vi "Autonomous Independent.vi"   [LabVIEW 2017]
doc: "This VI is called when autonomous begins, and will automatically be terminated when autonomous ends. You can carry out timed or sensor driven robot movement independently without needing to return to the caller."
uses:
  <vilib>/Rock Robotics/Network Tables/NT Read String.vi
  Robot Global Data.vi
  <vilib>/Rock Robotics/Network Tables/NT Write String.vi
  <vilib>/Rock Robotics/WPI/ThirdParty/Sensors/ADIS16448 IMU/ADIS16448_IMU.lvlib
types:
  T1 = typedef "ADIS16448_IMU.lvlib/ADI_IMU_ADIS16448_IMUDevRef.ctl" = cluster{"DevStatus":errorcluster, "Handle":i32, "SPI Bus":T2, "Device Found":bool, "Device Ready":bool, "Yaw Axis":enum16{"X", "Y", "Z"}, "AHRS Algorithm":enum16{"Complementary", "Madgwick"}, "Serial":u16, "Lot ID 2":u16, "Lot ID 1":u16, "Bytes Per Sample":u16, "Calibrate On Open?":bool}
  T2 = typedef "spi_bus.ctl" = enum16{"SPI On-Board, CS0", "SPI On-Board, CS1", "SPI On-Board, CS2", "SPI On-Board, CS3", "SPI MXP", "Invalid"}
  T3 = cluster{"X Angle":dbl, "Y Angle":dbl, "Z Angle":dbl}
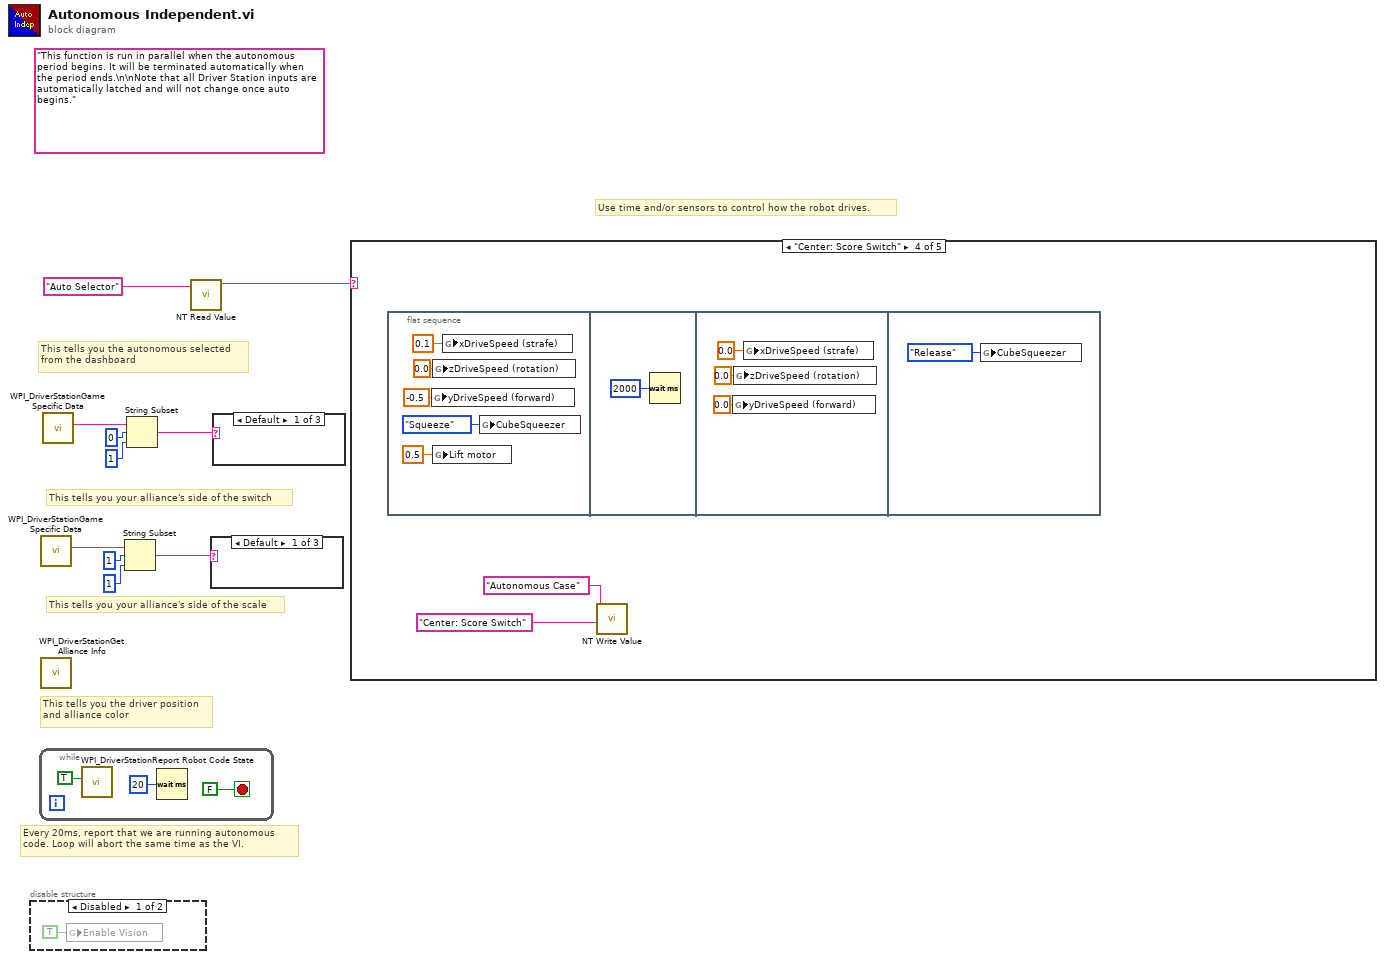
[diagram p0: block diagram]
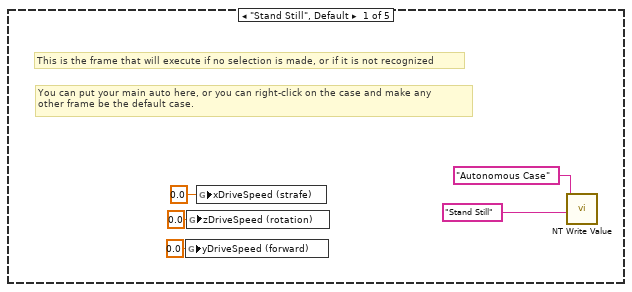
[diagram p7: hidden frame]
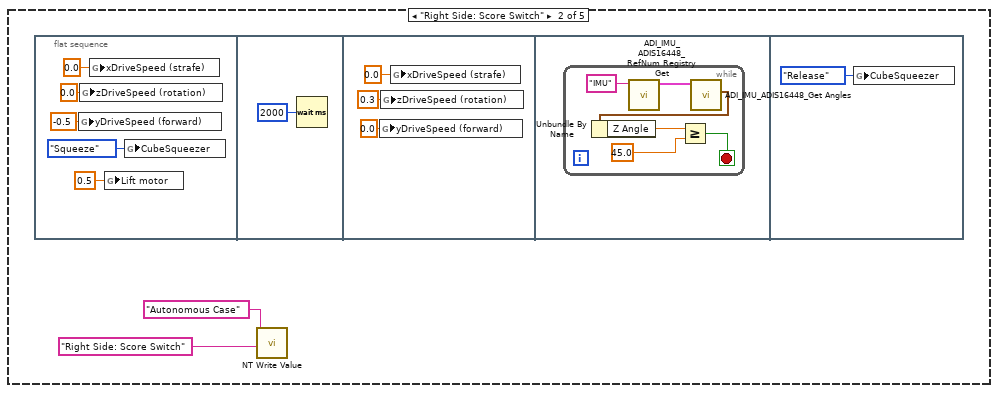
[diagram p8: hidden frame]
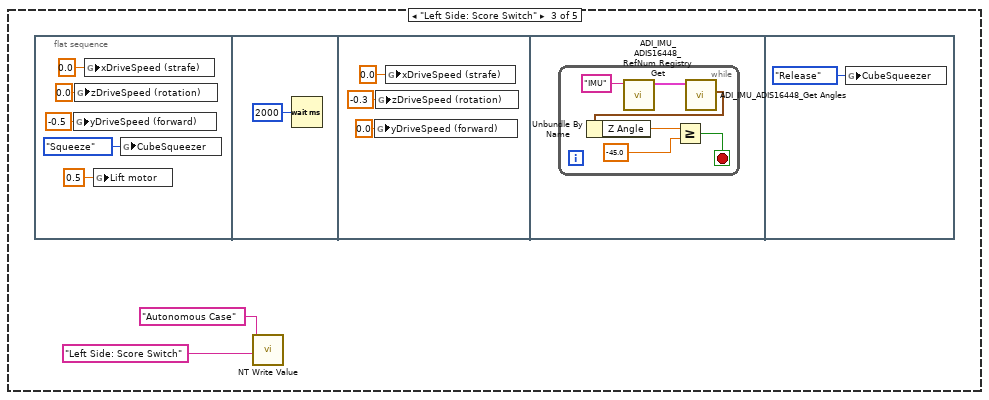
[diagram p9: hidden frame]
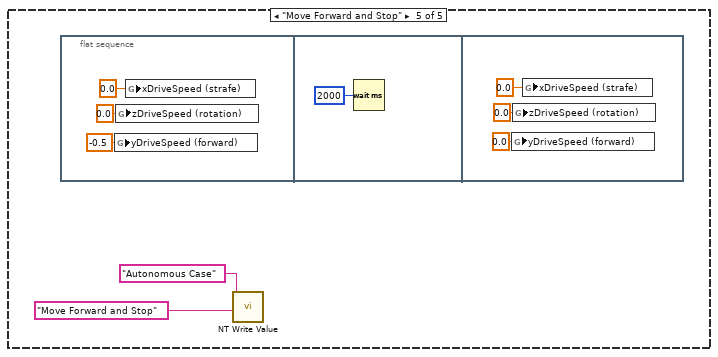
[diagram p10: hidden frame]
diagram:
  (unwired) "This function is run in parallel when the autonomous period begins. It will be terminated automatically when the period ends.\n\nNote that all Driver Station inputs are automatically latched and will not change once auto begins."
  # "This tells you your alliance's side of the scale"
  # "This tells you your alliance's side of the switch"
  # "This tells you the autonomous selected\nfrom the dashboard"
  # "Every 20ms, report that we are running autonomous\ncode. Loop will abort the same time as the VI."
  # "Use time and/or sensors to control how the robot drives."
  # "This tells you the driver position\nand alliance color"
  n1 = disable-structure shown="Disabled" {
    frame Disabled {
      n2 = global write "Robot Global Data.vi" "Enable Vision"(TRUE ("Enable Vision")) -> ()
    }
    frame Enabled {
    }
  }
  n3 = while {
    stop <- FALSE stop-if-true
    n4 = call <vilib>:"WPI_DriverStationReport Robot Code State.vi"("Autonomous"=TRUE) -> ()  [unwired: 10 in, 1 out]
    n5 = Wait (ms)(milliseconds to wait=u32 20) -> ()  [unwired: 1 out]
  }
  n6 = call <vilib>:"WPI_DriverStationGame Specific Data.vi"() -> ("Game Specific Data"=w5:string)  [unwired: 11 in]
  n7 = call <vilib>:"WPI_DriverStationGet Alliance Info.vi"() -> ()  [unwired: 12 out]
  n8 = call <vilib>:"WPI_DriverStationGame Specific Data.vi"() -> ("Game Specific Data"=w8:string)  [unwired: 11 in]
  n9 = String Subset(string=w5, offset (0)=1, length (rest)=1 ("length (rest)")) -> (substring=w3:string)
  n10 = String Subset(string=w8, offset (0)=0, length (rest)=1 ("length (rest)")) -> (substring=w6:string)
  n11 = call-poly <vilib>:"NT Read Value.vi"("Name"="Auto Selector") -> ("String"=w9:string)  [unwired: 9 in, 1 out]
  n12 = case shown="Default" w3 {
    frame Default {
    }
    frame "L" {
    }
    frame "R" {
    }
  }
  n13 = case shown="Default" w6 {
    frame Default {
    }
    frame "L" {
    }
    frame "R" {
    }
  }
  n14 = case shown="\"Center: Score Switch\"" w9 {
    frame "Stand Still", Default {
      # "You can put your main auto here, or you can right-click on the case and make any\nother frame be the default case."
      # "This is the frame that will execute if no selection is made, or if it is not recognized"
      n15 = global write "Robot Global Data.vi" "yDriveSpeed (forward)"(0.0 ("xDriveSpeed (strafe)")) -> ()
      n16 = global write "Robot Global Data.vi" "zDriveSpeed (rotation)"(0.0 ("xDriveSpeed (strafe)")) -> ()
      n17 = global write "Robot Global Data.vi" "xDriveSpeed (strafe)"(0.0 ("xDriveSpeed (strafe)")) -> ()
      n18 = call-poly <vilib>:"NT Write Value.vi"("String"="Stand Still", "Name"="Autonomous Case") -> ()  [unwired: 9 in, 1 out]
    }
    frame "Right Side: Score Switch" {
      n19 = flat-sequence {
        frame #0 {
          n20 = global write "Robot Global Data.vi" "yDriveSpeed (forward)"(-0.5 ("xDriveSpeed (strafe)")) -> ()
          n21 = global write "Robot Global Data.vi" "zDriveSpeed (rotation)"(0.0 ("xDriveSpeed (strafe)")) -> ()
          n22 = global write "Robot Global Data.vi" "xDriveSpeed (strafe)"(0.0 ("xDriveSpeed (strafe)")) -> ()
          n23 = global write "Robot Global Data.vi" "Lift motor"(0.5 ("Lift motor")) -> ()
          n24 = global write "Robot Global Data.vi" "CubeSqueezer"(enum16{"Squeeze", "Release"}."Squeeze" ("CubeSqueezer")) -> ()
        }
        frame #1 {
          n25 = Wait (ms)(milliseconds to wait=u32 2000) -> ()  [unwired: 1 out]
        }
        frame #2 {
          n26 = global write "Robot Global Data.vi" "yDriveSpeed (forward)"(0.0 ("xDriveSpeed (strafe)")) -> ()
          n27 = global write "Robot Global Data.vi" "zDriveSpeed (rotation)"(0.3 ("xDriveSpeed (strafe)")) -> ()
          n28 = global write "Robot Global Data.vi" "xDriveSpeed (strafe)"(0.0 ("xDriveSpeed (strafe)")) -> ()
        }
        frame #3 {
          n29 = while {
            stop <- w31 stop-if-true
            n30 = call <vilib>:"ADI_IMU_ADIS16448_RefNum Registry Get.vi"("refnum name"="IMU") -> ("ADI IMU DevRef"=w35:T1)  [unwired: 9 in, 1 out]
            n31 = call <vilib>:"ADI_IMU_ADIS16448_Get Angles.vi"("ADI IMU DevRef"=w35) -> ("IMU Angles Out"=w34:T3)  [unwired: 7 in, 3 out]
            n32 = Unbundle By Name(w34) -> ("Z Angle"=w33:dbl)
            n33 = Greater Or Equal?(x=w33, y=45.0) -> (x >= y?=w31:bool)
          }
        }
        frame #4 {
          n34 = global write "Robot Global Data.vi" "CubeSqueezer"(enum16{"Squeeze", "Release"}."Release" ("CubeSqueezer")) -> ()
        }
      }
      n35 = call-poly <vilib>:"NT Write Value.vi"("String"="Right Side: Score Switch", "Name"="Autonomous Case") -> ()  [unwired: 9 in, 1 out]
    }
    frame "Left Side: Score Switch" {
      n36 = flat-sequence {
        frame #0 {
          n37 = global write "Robot Global Data.vi" "yDriveSpeed (forward)"(-0.5 ("xDriveSpeed (strafe)")) -> ()
          n38 = global write "Robot Global Data.vi" "zDriveSpeed (rotation)"(0.0 ("xDriveSpeed (strafe)")) -> ()
          n39 = global write "Robot Global Data.vi" "xDriveSpeed (strafe)"(0.0 ("xDriveSpeed (strafe)")) -> ()
          n40 = global write "Robot Global Data.vi" "Lift motor"(0.5 ("Lift motor")) -> ()
          n41 = global write "Robot Global Data.vi" "CubeSqueezer"(enum16{"Squeeze", "Release"}."Squeeze" ("CubeSqueezer")) -> ()
        }
        frame #1 {
          n42 = Wait (ms)(milliseconds to wait=u32 2000) -> ()  [unwired: 1 out]
        }
        frame #2 {
          n43 = global write "Robot Global Data.vi" "yDriveSpeed (forward)"(0.0 ("xDriveSpeed (strafe)")) -> ()
          n44 = global write "Robot Global Data.vi" "zDriveSpeed (rotation)"(-0.3 ("xDriveSpeed (strafe)")) -> ()
          n45 = global write "Robot Global Data.vi" "xDriveSpeed (strafe)"(0.0 ("xDriveSpeed (strafe)")) -> ()
        }
        frame #3 {
          n46 = while {
            stop <- w49 stop-if-true
            n47 = call <vilib>:"ADI_IMU_ADIS16448_RefNum Registry Get.vi"("refnum name"="IMU") -> ("ADI IMU DevRef"=w53:T1)  [unwired: 9 in, 1 out]
            n48 = call <vilib>:"ADI_IMU_ADIS16448_Get Angles.vi"("ADI IMU DevRef"=w53) -> ("IMU Angles Out"=w52:T3)  [unwired: 7 in, 3 out]
            n49 = Unbundle By Name(w52) -> ("Z Angle"=w51:dbl)
            n50 = Greater Or Equal?(x=w51, y=-45.0) -> (x >= y?=w49:bool)
          }
        }
        frame #4 {
          n51 = global write "Robot Global Data.vi" "CubeSqueezer"(enum16{"Squeeze", "Release"}."Release" ("CubeSqueezer")) -> ()
        }
      }
      n52 = call-poly <vilib>:"NT Write Value.vi"("String"="Left Side: Score Switch", "Name"="Autonomous Case") -> ()  [unwired: 9 in, 1 out]
    }
    frame "Center: Score Switch" {
      n53 = flat-sequence {
        frame #0 {
          n54 = global write "Robot Global Data.vi" "yDriveSpeed (forward)"(-0.5 ("xDriveSpeed (strafe)")) -> ()
          n55 = global write "Robot Global Data.vi" "zDriveSpeed (rotation)"(0.0 ("xDriveSpeed (strafe)")) -> ()
          n56 = global write "Robot Global Data.vi" "Lift motor"(0.5 ("Lift motor")) -> ()
          n57 = global write "Robot Global Data.vi" "xDriveSpeed (strafe)"(0.1 ("xDriveSpeed (strafe)")) -> ()
          n58 = global write "Robot Global Data.vi" "CubeSqueezer"(enum16{"Squeeze", "Release"}."Squeeze" ("CubeSqueezer")) -> ()
        }
        frame #1 {
          n59 = Wait (ms)(milliseconds to wait=u32 2000) -> ()  [unwired: 1 out]
        }
        frame #2 {
          n60 = global write "Robot Global Data.vi" "yDriveSpeed (forward)"(0.0 ("xDriveSpeed (strafe)")) -> ()
          n61 = global write "Robot Global Data.vi" "zDriveSpeed (rotation)"(0.0 ("xDriveSpeed (strafe)")) -> ()
          n62 = global write "Robot Global Data.vi" "xDriveSpeed (strafe)"(0.0 ("xDriveSpeed (strafe)")) -> ()
        }
        frame #3 {
          n63 = global write "Robot Global Data.vi" "CubeSqueezer"(enum16{"Squeeze", "Release"}."Release" ("CubeSqueezer")) -> ()
        }
      }
      n64 = call-poly <vilib>:"NT Write Value.vi"("String"="Center: Score Switch", "Name"="Autonomous Case") -> ()  [unwired: 9 in, 1 out]
    }
    frame "Move Forward and Stop" {
      n65 = flat-sequence {
        frame #0 {
          n66 = global write "Robot Global Data.vi" "yDriveSpeed (forward)"(-0.5 ("xDriveSpeed (strafe)")) -> ()
          n67 = global write "Robot Global Data.vi" "zDriveSpeed (rotation)"(0.0 ("xDriveSpeed (strafe)")) -> ()
          n68 = global write "Robot Global Data.vi" "xDriveSpeed (strafe)"(0.0 ("xDriveSpeed (strafe)")) -> ()
        }
        frame #1 {
          n69 = Wait (ms)(milliseconds to wait=u32 2000) -> ()  [unwired: 1 out]
        }
        frame #2 {
          n70 = global write "Robot Global Data.vi" "yDriveSpeed (forward)"(0.0 ("xDriveSpeed (strafe)")) -> ()
          n71 = global write "Robot Global Data.vi" "zDriveSpeed (rotation)"(0.0 ("xDriveSpeed (strafe)")) -> ()
          n72 = global write "Robot Global Data.vi" "xDriveSpeed (strafe)"(0.0 ("xDriveSpeed (strafe)")) -> ()
        }
      }
      n73 = call-poly <vilib>:"NT Write Value.vi"("String"="Move Forward and Stop", "Name"="Autonomous Case") -> ()  [unwired: 9 in, 1 out]
    }
  }
